vi "Gravity.vi"() -> ()   [LabVIEW 2013]
panel:
  out "Gravity":dbl
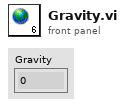
[diagram p1: front panel]
diagram:
